vi "Configure List Terminate Type.vi"(8 "error in":errorcluster, 10 "Terminate Type":u16(ring) items=["Normal", "Last"], 11 "VISA resource name":refnum<visa-resource-name>) -> (0 "error out":errorcluster, 3 "VISA resource name out":refnum<visa-resource-name>)   [LabVIEW 2018, in "IT-M3100.lvlib"]
doc: "This command sets the end state of the list program.\n<b>Terminate Type</b>\n0:Normal\n1:Last"
uses:
  IT-M3100.lvlib
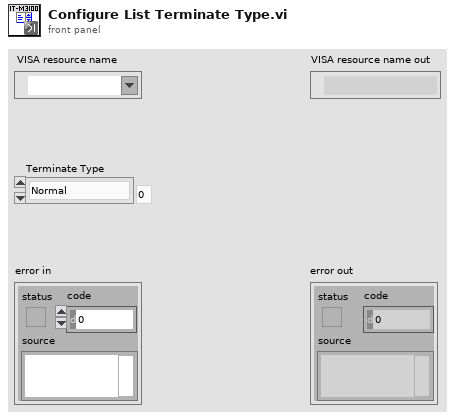
[diagram p1: front panel]
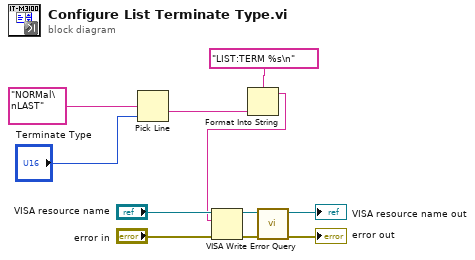
[diagram p0: block diagram]
diagram:
  n1 = Pick Line(multi-line string="NORMal\nLAST", line index="Terminate Type") -> (output string=w2:string)  [unwired: 1 in]
  n2 = Format Into String(format string="LIST:TERM %s\n", w2) -> (resulting string=w1:string)  [unwired: 2 in, 1 out]
  n3 = VISA Write(VISA resource name="VISA resource name", write buffer=w1, error in (no error)="error in") -> (VISA resource name out=w8:refnum<visa-resource-name>, error out=w9:errorcluster)  [unwired: 1 out]
  n4 = call "Error Query.vi"("error in"=w9, "VISA resource name"=w8) -> ("error out"=→"error out":errorcluster, "VISA resource name out"=→"VISA resource name out":refnum<visa-resource-name>)  [unwired: 6 in, 2 out]
